vi "Short Circuit Impedance.vi"(0 "one-cycle fundamental voltage vectors":T2(array[cluster]), 1 "reset? (F)":bool, 5 "one-cycle fundamental current vectors":T2(array[cluster]), 9 "system info in":refnum<class "EP System Info.lvclass">, 11 "error in (no error)":errorcluster) -> (4 "short impedance":cdb[](array[numeric]), 10 "system info out":refnum<class "EP System Info.lvclass">, 15 "error out":errorcluster)   [LabVIEW 2012, in "NI_EP_Power Quality.lvlib"]
doc: "Calculates the short-circuit impedance. You can use the <b>EP D to Y Conversion</b> VI to calculate the <b>one period fundamental voltage vectors</b>."
uses:
  <vilib>/addons/Electrical Power/PQ/NI_EP_Power Quality.lvlib
  <vilib>/addons/Electrical Power/PQ/Common/Controls/ep_AI Data Channel.ctl
  <vilib>/addons/Electrical Power/PQ/Common/Classes/System Info/EP System Info.lvclass
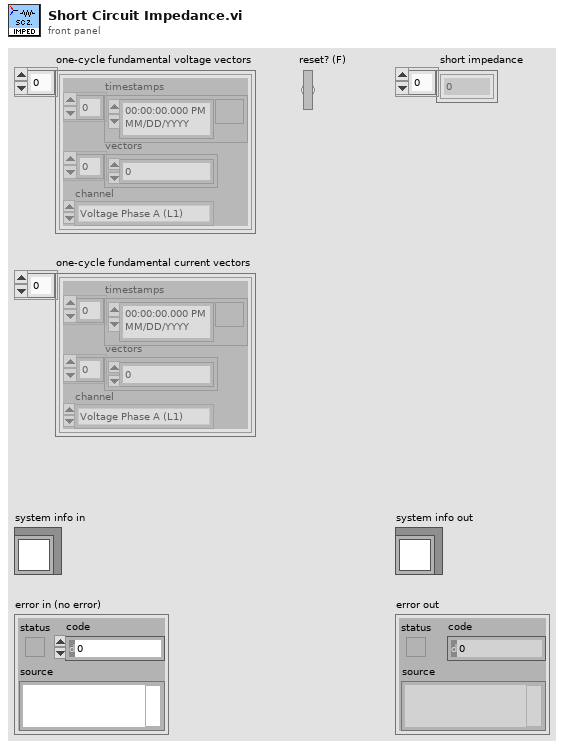
[diagram p1: front panel]
types:
  T1 = typedef "NI_EP_Power Quality.lvlib/ep_AI Data Channel.ctl" = enum16{"Voltage Phase A (L1)", "Voltage Phase B (L2)", "Voltage Phase C (L3)", "Voltage Phase N (Neutral)", "Current Phase A (L1)", "Current Phase B (L2)", "Current Phase C (L3)", "Current Phase N (Neutral)"}
  T2 = cluster{"timestamps":timestamp[], "vectors":cdb[], "channel":T1}[]
  T3 = cluster{"timestamps":timestamp[], "vectors":cdb[], "channel":T1}
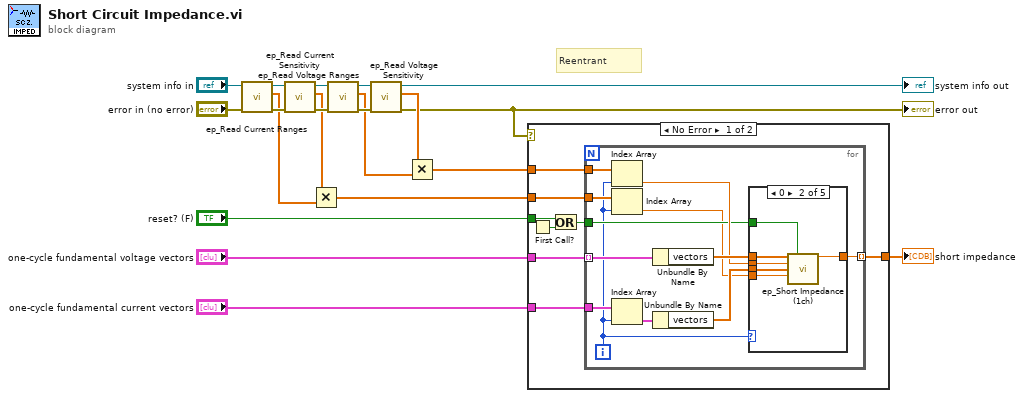
[diagram p0: block diagram]
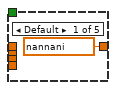
[diagram p2: hidden frame]
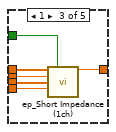
[diagram p3: hidden frame]
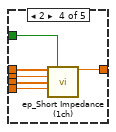
[diagram p4: hidden frame]
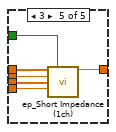
[diagram p5: hidden frame]
diagram:
  # "Reentrant"
  n1 = call <vilib>:"ep_Read Current Ranges.vi"("error in (no error)"="error in (no error)", "system info in"="system info in") -> ("error out"=w17:errorcluster, "current ranges"=w13:dbl[], "system info out"=w20:refnum<class "EP System Info.lvclass">)  [unwired: 7 in]
  n2 = call <vilib>:"ep_Read Current Sensitivity.vi"("error in (no error)"=w17, "system info in"=w20) -> ("error out"=w16:errorcluster, "current sensitivity"=w14:dbl[], "system info out"=w19:refnum<class "EP System Info.lvclass">)  [unwired: 7 in]
  n3 = Multiply(x=w14, y=w13) -> (x*y=w9:dbl[])
  n4 = call <vilib>:"ep_Read Voltage Ranges.vi"("error in (no error)"=w16, "system info in"=w19) -> ("error out"=w15:errorcluster, "voltage ranges"=w11:dbl[], "system info out"=w18:refnum<class "EP System Info.lvclass">)  [unwired: 7 in]
  n5 = call <vilib>:"ep_Read Voltage Sensitivity.vi"("error in (no error)"=w15, "system info in"=w18) -> ("error out"=w2:errorcluster, "voltage sensitivity"=w12:dbl[], "system info out"=→"system info out":refnum<class "EP System Info.lvclass">)  [unwired: 7 in]
  "error out" <- w2
  n6 = Multiply(x=w12, y=w11) -> (x*y=w10:dbl[])
  n7 = case shown="No Error" w2 {
    tunnel: "one-cycle fundamental voltage vectors" -> [w27 _]
    tunnel: "one-cycle fundamental current vectors" -> [w24 _]
    tunnel: w10 -> [w26 _]
    tunnel: w9 -> [w25 _]
    tunnel: [w28 _] -> w8
    tunnel: "reset? (F)" -> [w22 _]
    frame No Error {
      n8 = First Call?() -> (First Call?: T/F=w23:bool)
      n9 = Or(x=w22, y=w23) -> (x .or. y?=w21:bool)
      n10 = for {
        tunnel: w27 -> [w40] mode=indexing
        tunnel: w24 -> [w33]
        tunnel: w25 -> [w34]
        tunnel: w26 -> [w36]
        tunnel: [w39] -> w28 mode=indexing
        tunnel: w21 -> [w31]
        i -> [w29]
        n11 = Index Array(array=w36, index=w29) -> (element=w35:dbl)
        n12 = Index Array(array=w34, index=w29) -> (element=w30:dbl)
        n13 = Index Array(array=w33, index=w29) -> (element=w32:T3)
        n14 = Unbundle By Name(w40) -> ("vectors"=w38:cdb[])
        n15 = Unbundle By Name(w32) -> ("vectors"=w37:cdb[])
        n16 = case shown="0" w29 {
          tunnel: w35 -> [_ w45 w51 w57 w63]
          tunnel: [cdb nan+nani ("mean") w43 w49 w55 w61] -> w39
          tunnel: w38 -> [_ w47 w53 w59 w65]
          tunnel: w37 -> [_ w46 w52 w58 w64]
          tunnel: w30 -> [_ w44 w50 w56 w62]
          tunnel: w31 -> [_ w42 w48 w54 w60]
          frame Default {
          }
          frame 0 {
            n17 = call <vilib>:"ep_Short Impedance (1ch).vi"("fundamental voltage vectors"=w47, "restart (F)"=w42, "voltage range*sensitivity"=w45, "fundamental current vectors"=w46, "current range*sensitivity"=w44) -> ("short impedance"=w43:cdb)  [unwired: 10 in]
          }
          frame 1 {
            n18 = call <vilib>:"ep_Short Impedance (1ch).vi"("fundamental voltage vectors"=w53, "restart (F)"=w48, "voltage range*sensitivity"=w51, "fundamental current vectors"=w52, "current range*sensitivity"=w50) -> ("short impedance"=w49:cdb)  [unwired: 10 in]
          }
          frame 2 {
            n19 = call <vilib>:"ep_Short Impedance (1ch).vi"("fundamental voltage vectors"=w59, "restart (F)"=w54, "voltage range*sensitivity"=w57, "fundamental current vectors"=w58, "current range*sensitivity"=w56) -> ("short impedance"=w55:cdb)  [unwired: 10 in]
          }
          frame 3 {
            n20 = call <vilib>:"ep_Short Impedance (1ch).vi"("fundamental voltage vectors"=w65, "restart (F)"=w60, "voltage range*sensitivity"=w63, "fundamental current vectors"=w64, "current range*sensitivity"=w62) -> ("short impedance"=w61:cdb)  [unwired: 10 in]
          }
        }
      }
    }
    frame Error {
    }
  }
  "short impedance" <- w8
